vi "ZeroMQ_GS.vi"() -> ()   [LabVIEW 2018]
uses:
  <vilib>/addons/zeromq/socket_type.ctl
  <vilib>/addons/zeromq/socket_options.ctl
  <vilib>/addons/zeromq/zeromq.lvlib
  <vilib>/addons/zeromq/zmq_socket.lvclass
  <vilib>/addons/zeromq/zmq_context.lvclass
panel:
  in  "Cluster":T1
  out "command":string
  in  "stop 3":bool
  out "error out 3":errorcluster
  out "pub":string
  out "error out 2":errorcluster
  out "sub":string
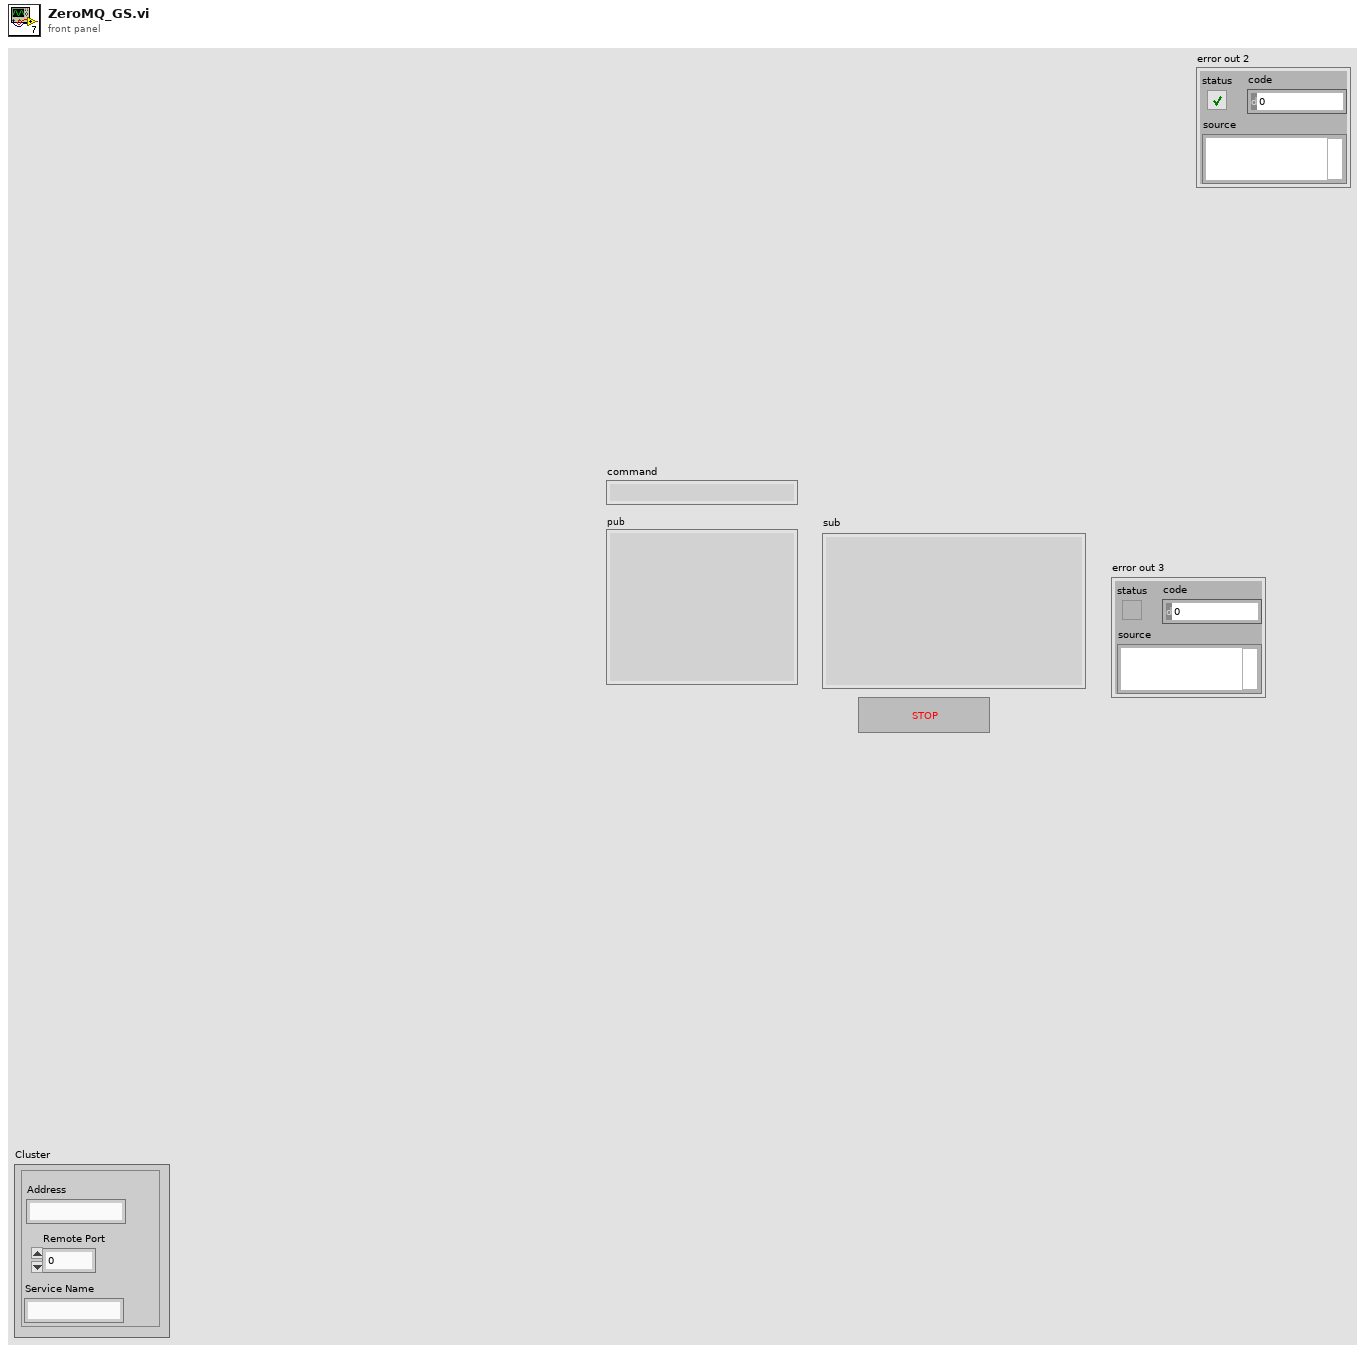
[diagram p1: front panel]
types:
  T1 = cluster{"Address":string, "Remote Port":u32, "Service Name":string}
  T2 = typedef "zeromq.lvlib/socket_type.ctl" = enum8{"ZMQ_PAIR", "ZMQ_PUB", "ZMQ_SUB", "ZMQ_REQ", "ZMQ_REP", "ZMQ_DEALER", "ZMQ_ROUTER", "ZMQ_PULL", "ZMQ_PUSH", "ZMQ_XPUB", "ZMQ_XSUB", "ZMQ_STREAM", "ZMQ_SERVER", "ZMQ_CLIENT", "ZMQ_RADIO", "ZMQ_DISH", "ZMQ_GATHER", "ZMQ_SCATTER", "ZMQ_DGRAM"}
  T3 = typedef "zeromq.lvlib/socket_options.ctl" = enum8{"NONE", "ZMQ_HWM", "<2>", "ZMQ_SWAP", "ZMQ_AFFINITY", "ZMQ_ROUTING_ID", "ZMQ_SUBSCRIBE", "ZMQ_UNSUBSCRIBE", "ZMQ_RATE", "ZMQ_RECOVERY_IVL", "ZMQ_MCAST_LOOP", "ZMQ_SNDBUF", "ZMQ_RCVBUF", "ZMQ_RCVMORE", "ZMQ_FD", "ZMQ_EVENTS", "ZMQ_TYPE", "ZMQ_LINGER", "ZMQ_RECONNECT_IVL", "ZMQ_BACKLOG", "ZMQ_RECOVERY_IVL_MSEC", "ZMQ_RECONNECT_IVL_MAX", "ZMQ_MAXMSGSIZE", "ZMQ_SNDHWM", "ZMQ_RCVHWM", "ZMQ_MULTICAST_HOPS", "<26>", "ZMQ_RCVTIMEO", "ZMQ_SNDTIMEO", "<29>", "<30>", "ZMQ_IPV4ONLY", "ZMQ_LAST_ENDPOINT", "ZMQ_ROUTER_MANDATORY", "ZMQ_TCP_KEEPALIVE", "ZMQ_TCP_KEEPALIVE_CNT", "ZMQ_TCP_KEEPALIVE_IDLE", "ZMQ_TCP_KEEPALIVE_INTVL", "ZMQ_TCP_ACCEPT_FILTER", "ZMQ_IMMEDIATE", "ZMQ_XPUB_VERBOSE", "ZMQ_ROUTER_RAW", "ZMQ_IPV6", "ZMQ_MECHANISM", "ZMQ_PLAIN_SERVER", "ZMQ_PLAIN_USERNAME", "ZMQ_PLAIN_PASSWORD", "ZMQ_CURVE_SERVER", "ZMQ_CURVE_PUBLICKEY", "ZMQ_CURVE_SECRETKEY", "ZMQ_CURVE_SERVERKEY", "ZMQ_PROBE_ROUTER", "ZMQ_REQ_CORRELATE", "ZMQ_REQ_RELAXED", "ZMQ_CONFLATE", "ZMQ_ZAP_DOMAIN", "ZMQ_ROUTER_HANDOVER", "ZMQ_TOS", "ZMQ_IPC_FILTER_PID", "ZMQ_IPC_FILTER_UID", "ZMQ_IPC_FILTER_GID", "ZMQ_CONNECT_ROUTING_ID", "ZMQ_GSSAPI_SERVER", "ZMQ_GSSAPI_PRINCIPAL", "ZMQ_GSSAPI_SERVICE_PRINCIPAL", "ZMQ_GSSAPI_PLAINTEXT", "ZMQ_HANDSHAKE_IVL", "<67>", "ZMQ_SOCKS_PROXY", "ZMQ_XPUB_NODROP", "ZMQ_BLOCKY", "ZMQ_XPUB_MANUAL", "ZMQ_XPUB_WELCOME_MSG", "ZMQ_STREAM_NOTIFY", "ZMQ_INVERT_MATCHING", "ZMQ_HEARTBEAT_IVL", "ZMQ_HEARTBEAT_TTL", "ZMQ_HEARTBEAT_TIMEOUT", "ZMQ_XPUB_VERBOSER", "ZMQ_CONNECT_TIMEOUT", "ZMQ_TCP_MAXRT", "ZMQ_THREAD_SAFE", "<82>", "<83>", "ZMQ_MULTICAST_MAXTPDU", "ZMQ_VMCI_BUFFER_SIZE", "ZMQ_VMCI_BUFFER_MIN_SIZE", "ZMQ_VMCI_BUFFER_MAX_SIZE", "ZMQ_VMCI_CONNECT_TIMEOUT", "ZMQ_USE_FD", "ZMQ_GSSAPI_PRINCIPAL_NAMETYPE", "ZMQ_GSSAPI_SERVICE_PRINCIPAL_NAMETYPE", "ZMQ_BINDTODEVICE", "ZMQ_ZAP_ENFORCE_DOMAIN", "ZMQ_LOOPBACK_FASTPATH", "ZMQ_METADATA", "ZMQ_MULTICAST_LOOP", "ZMQ_ROUTER_NOTIFY"}
  T4 = cluster{"ID":u32, "Address":string, "Service Name 1":string, "Service Name 2":string, "queue TX":refnum<queue>, "queue RX":refnum<queue>, "Port 1":u32, "Port 2":u32}
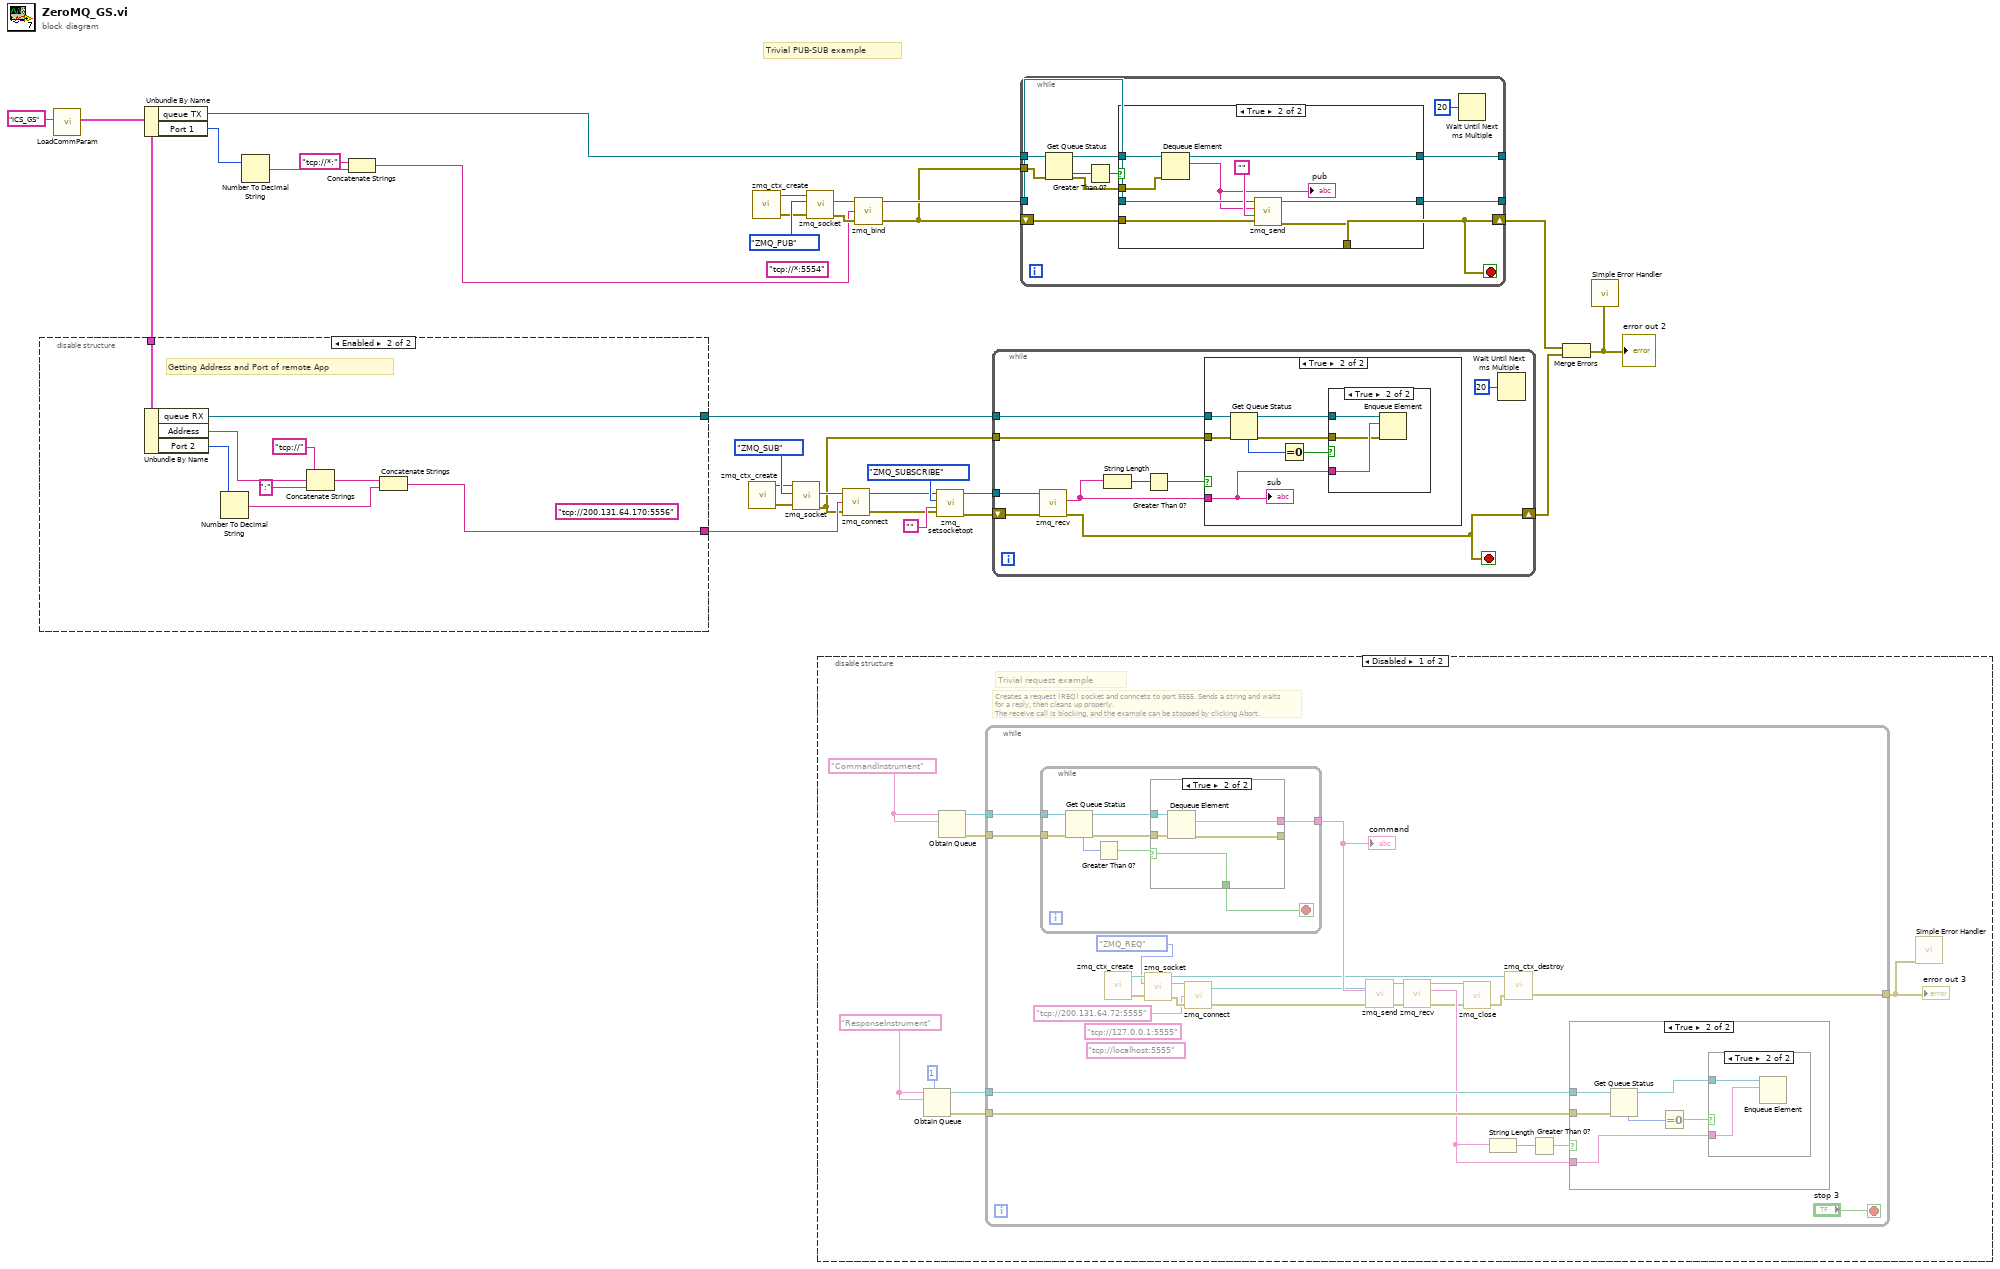
[diagram p0: block diagram]
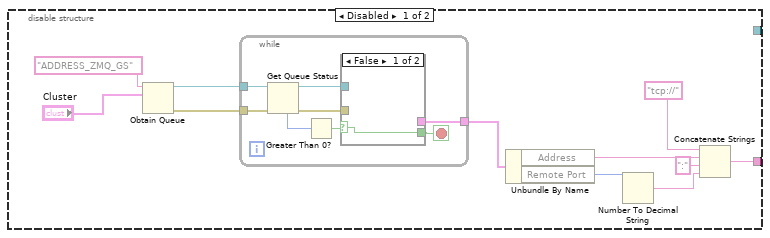
[diagram p2: hidden frame]
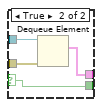
[diagram p3: hidden frame]
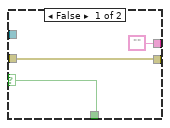
[diagram p9: hidden frame]
diagram:
  (unwired) "tcp://*:5554" ("endpoint")
  # "Trivial PUB-SUB example"
  n1 = call "LoadCommParam.vi"("section name"="ICS_GS") -> ("output cluster"=w3:T4)  [unwired: 10 in]
  n2 = disable-structure shown="Enabled" {
    disable-tunnel: [w31 w55] -> w11
    disable-tunnel: w3 -> [_ w57]
    disable-tunnel: [_ w56] -> w1
    frame Disabled {
      n3 = Obtain Queue(name (unnamed)="ADDRESS_ZMQ_GS", element data type="Cluster") -> (queue out=w39:refnum<queue>, error out=w40:errorcluster)  [unwired: 3 in, 1 out]
      n4 = while {
        tunnel: [w49] -> w37
        tunnel: w40 -> [w47]
        tunnel: w39 -> [w46]
        stop <- w42 stop-if-true
        n5 = Get Queue Status(queue=w46, error in (no error)=w47) -> (queue out=w45:refnum<queue>, error out=w48:errorcluster, # elements in queue=w44:i32)  [unwired: 1 in, 5 out]
        n6 = Greater Than 0?(x=w44) -> (x > 0?=w43:bool)
        n7 = case shown="False" w43 {
          selector: w43 -> [w50 w51]
          tunnel: [_ w54] -> w49
          tunnel: w48 -> [_ w53]
          tunnel: w45 -> [_ w52]
          tunnel: [w50 w51] -> w42
          frame False {
          }
          frame True {
            n8 = Dequeue Element(queue=w52, error in (no error)=w53) -> (element=w54:T1)  [unwired: 1 in, 3 out]
          }
        }
      }
      n9 = Unbundle By Name(w37) -> ("Address"=w35:string, "Remote Port"=w34:u32)
      n10 = Number To Decimal String(number=w34) -> (decimal integer string=w33:string)  [unwired: 1 in]
      n11 = Concatenate Strings("tcp://" ("string"), w35, ":" ("string"), w33) -> (w31:string)
    }
    frame Enabled {
      (unwired) "tcp://200.131.64.170:5556" ("endpoint")
      # "Getting Address and Port of remote App"
      n12 = Unbundle By Name(w57) -> ("queue RX"=w56:refnum<queue>, "Address"=w60:string, "Port 2"=w61:u32)
      n13 = Number To Decimal String(number=w61) -> (decimal integer string=w62:string)  [unwired: 1 in]
      n14 = Concatenate Strings("tcp://" ("string"), w60, ":" ("string")) -> (w63:string)
      n15 = Concatenate Strings(w63, w62) -> (w55:string)
    }
  }
  n16 = Unbundle By Name(w3) -> ("queue TX"=w7:refnum<queue>, "Port 1"=w9:u32)
  n17 = Number To Decimal String(number=w9) -> (decimal integer string=w8:string)  [unwired: 1 in]
  n18 = Concatenate Strings("tcp://*:" ("string"), w8) -> (w4:string)
  n19 = call <vilib>:"zmq_ctx_create.vi"() -> ("error out"=w29:errorcluster, "context out"=w15:refnum<class "zmq_context.lvclass">)  [unwired: 4 in]
  n20 = call <vilib>:"zmq_ctx_create.vi"() -> ("error out"=w20:errorcluster, "context out"=w23:refnum<class "zmq_context.lvclass">)  [unwired: 4 in]
  n21 = call <vilib>:"zmq_socket.vi"("error in"=w29, "socket type"=socket_type."ZMQ_SUB", "context in"=w15) -> ("error out"=w2:errorcluster, "socket out"=w24:refnum<class "zmq_socket.lvclass">)  [unwired: 2 in, 1 out]
  n22 = call <vilib>:"zmq_socket.vi"("error in"=w20, "socket type"=socket_type."ZMQ_PUB", "context in"=w23) -> ("error out"=w19:errorcluster, "socket out"=w21:refnum<class "zmq_socket.lvclass">)  [unwired: 2 in, 1 out]
  n23 = disable-structure shown="Disabled" {
    frame Disabled {
      w64 = "ResponseInstrument"
      w65 = "CommandInstrument"
      # "Creates a request (REQ) socket and conncets to port 5555. Sends a string and waits for a reply, then cleans up properly.\nThe receive call is blocking, and the example can be stopped by clicking Abort."
      # "Trivial request example"
      n24 = Obtain Queue(max queue size (-1, unlimited)=1, name (unnamed)=w64, element data type=w64) -> (queue out=w68:refnum<queue>, error out=w67:errorcluster)  [unwired: 2 in, 1 out]
      n25 = Obtain Queue(name (unnamed)=w65, element data type=w65) -> (queue out=w70:refnum<queue>, error out=w69:errorcluster)  [unwired: 3 in, 1 out]
      n26 = while {
        tunnel: w70 -> [w93]
        tunnel: w69 -> [w92]
        tunnel: w68 -> [w90]
        tunnel: w67 -> [w89]
        tunnel: [w76] -> w66
        stop <- "stop 3" stop-if-true
        (unwired) "tcp://127.0.0.1:5555" ("endpoint")
        (unwired) "tcp://localhost:5555" ("endpoint")
        n27 = while {
          tunnel: w93 -> [w110]
          tunnel: w92 -> [w109]
          tunnel: [w105] -> w91
          stop <- w104 stop-if-true
          n28 = Get Queue Status(queue=w110, error in (no error)=w109) -> (queue out=w106:refnum<queue>, error out=w107:errorcluster, # elements in queue=w111:i32)  [unwired: 1 in, 5 out]
          n29 = Greater Than 0?(x=w111) -> (x > 0?=w108:bool)
          n30 = case shown="True" w108 {
            selector: w108 -> [w112 w115]
            tunnel: w107 -> [w114 w119]
            tunnel: w106 -> [_ w118]
            tunnel: [w114 w117] -> _
            tunnel: ["" w116] -> w105
            tunnel: [w112 w115] -> w104
            frame False {
            }
            frame True {
              n31 = Dequeue Element(queue=w118, error in (no error)=w119) -> (element=w116:string, error out=w117:errorcluster)  [unwired: 1 in, 2 out]
            }
          }
        }
        "command" <- w91
        n32 = call <vilib>:"zmq_ctx_create.vi"() -> ("error out"=w81:errorcluster, "context out"=w84:refnum<class "zmq_context.lvclass">)  [unwired: 4 in]
        n33 = call <vilib>:"zmq_socket.vi"("error in"=w81, "socket type"=socket_type."ZMQ_REQ", "context in"=w84) -> ("error out"=w83:errorcluster, "socket out"=w82:refnum<class "zmq_socket.lvclass">, "context out"=w73:refnum<class "zmq_context.lvclass">)  [unwired: 2 in]
        n34 = call <vilib>:"zmq_connect.vi"("error in"=w83, "endpoint"="tcp://200.131.64.72:5555", "socket in"=w82) -> ("error out"=w78:errorcluster, "socket out"=w79:refnum<class "zmq_socket.lvclass">)  [unwired: 1 in]
        n35 = call <vilib>:"zmq_send.vi"("error in"=w78, "data"=w91, "socket in"=w79) -> ("error out"=w94:errorcluster, "socket out"=w95:refnum<class "zmq_socket.lvclass">)  [unwired: 4 in]
        n36 = call <vilib>:"zmq_recv.vi"("error in"=w94, "socket in"=w95) -> ("error out"=w75:errorcluster, "data"=w87:string, "socket out"=w74:refnum<class "zmq_socket.lvclass">)  [unwired: 3 in, 2 out]
        n37 = call <vilib>:"zmq_close.vi"("error in"=w75, "socket"=w74) -> ("error out"=w77:errorcluster)  [unwired: 3 in]
        n38 = String Length(string=w87) -> (length=w88:i32)
        n39 = call <vilib>:"zmq_ctx_destroy.vi"("error in"=w77, "context in"=w73) -> ("error out"=w76:errorcluster)  [unwired: 3 in]
        n40 = Greater Than 0?(x=w88) -> (x > 0?=w86:bool)
        n41 = case shown="True" w86 {
          tunnel: w90 -> [_ w100]
          tunnel: w87 -> [_ w97]
          tunnel: w89 -> [_ w96]
          frame False {
          }
          frame True {
            n42 = Get Queue Status(queue=w100, error in (no error)=w96) -> (queue out=w98:refnum<queue>, # elements in queue=w101:i32)  [unwired: 1 in, 6 out]
            n43 = Equal To 0?(x=w101) -> (x = 0?=w99:bool)
            n44 = case shown="True" w99 {
              tunnel: w98 -> [_ w103]
              tunnel: w97 -> [_ w102]
              frame False {
              }
              frame True {
                n45 = Enqueue Element(queue=w103, element=w102) -> ()  [unwired: 2 in, 3 out]
              }
            }
          }
        }
      }
      "error out 3" <- w66
      n46 = call <vilib>:"Simple Error Handler.vi"("error in (no error)"=w66) -> ()  [unwired: 4 in, 5 out]
    }
    frame Enabled {
    }
  }
  n47 = call <vilib>:"zmq_connect.vi"("error in"=w2, "endpoint"=w11, "socket in"=w24) -> ("error out"=w13:errorcluster, "socket out"=w14:refnum<class "zmq_socket.lvclass">)  [unwired: 1 in]
  n48 = call <vilib>:"zmq_bind.vi"("error in"=w19, "endpoint"=w4, "socket in"=w21) -> ("error out"=w6:errorcluster, "socket out"=w12:refnum<class "zmq_socket.lvclass">)  [unwired: 1 in]
  n49 = call <vilib>:"zmq_setsocketopt.vi"("error in"=w13, "value"="", "option"=socket_options."ZMQ_SUBSCRIBE", "socket in"=w14) -> ("error out"=w28:errorcluster, "socket out"=w27:refnum<class "zmq_socket.lvclass">)  [unwired: 2 in]
  n50 = while {
    tunnel: w27 -> [w121]
    tunnel: w1 -> [w124]
    shift-right: [w127] -> w17
    shift-left: w28 -> [w128]
    tunnel: w2 -> [w122]
    stop <- w127 stop-if-true
    n51 = call <vilib>:"zmq_recv.vi"("error in"=w128, "socket in"=w121) -> ("error out"=w127:errorcluster, "data"=w123:string)  [unwired: 3 in, 3 out]
    n52 = String Length(string=w123) -> (length=w126:i32)
    n53 = Greater Than 0?(x=w126) -> (x > 0?=w125:bool)
    n54 = case shown="True" w125 {
      tunnel: w124 -> [_ w134]
      tunnel: w123 -> [_ w131]
      tunnel: w122 -> [_ w130]
      frame False {
      }
      frame True {
        n55 = Get Queue Status(queue=w134, error in (no error)=w130) -> (queue out=w132:refnum<queue>, error out=w129:errorcluster, # elements in queue=w135:i32)  [unwired: 1 in, 5 out]
        n56 = Equal To 0?(x=w135) -> (x = 0?=w133:bool)
        n57 = case shown="True" w133 {
          tunnel: w132 -> [_ w138]
          tunnel: w131 -> [_ w137]
          tunnel: w129 -> [_ w136]
          frame False {
          }
          frame True {
            n58 = Enqueue Element(queue=w138, element=w137, error in (no error)=w136) -> ()  [unwired: 1 in, 3 out]
          }
        }
        "sub" <- w131
      }
    }
    n59 = Wait Until Next ms Multiple(millisecond multiple=u32 20) -> ()  [unwired: 1 out]
  }
  n60 = while {
    tunnel: w12 -> [w146]
    tunnel: w7 -> [w150]
    tunnel: [w144] -> _
    tunnel: [w145] -> _
    tunnel: w6 -> [w143]
    shift-right: [w140] -> w18
    shift-left: w6 -> [w141]
    stop <- w140 stop-if-true
    n61 = Get Queue Status(queue=w150, error in (no error)=w143) -> (queue out=w149:refnum<queue>, error out=w142:errorcluster, # elements in queue=w148:i32)  [unwired: 1 in, 5 out]
    n62 = Greater Than 0?(x=w148) -> (x > 0?=w147:bool)
    n63 = case shown="True" w147 {
      tunnel: w149 -> [w152 w162]
      tunnel: w146 -> [w153 w160]
      tunnel: [w153 w158] -> w145
      tunnel: [w152 w159] -> w144
      tunnel: w142 -> [w151 w157]
      tunnel: [w151 w155] -> w140
      tunnel: w141 -> [_ w156]
      frame False {
      }
      frame True {
        n64 = Dequeue Element(queue=w162, error in (no error)=w157) -> (queue out=w159:refnum<queue>, element=w154:string)  [unwired: 1 in, 2 out]
        "pub" <- w154
        n65 = call <vilib>:"zmq_send.vi"("error in"=w156, "group"="", "data"=w154, "socket in"=w160) -> ("error out"=w155:errorcluster, "socket out"=w158:refnum<class "zmq_socket.lvclass">)  [unwired: 3 in]
      }
    }
    n66 = Wait Until Next ms Multiple(millisecond multiple=u32 20) -> ()  [unwired: 1 out]
  }
  n67 = Merge Errors(w18, w17) -> (w16:errorcluster)
  "error out 2" <- w16
  n68 = call <vilib>:"Simple Error Handler.vi"("error in (no error)"=w16) -> ()  [unwired: 4 in, 5 out]
